vi "Run Rx - New Data.vi"(7 "New Data Support in":T1, 8 "error in (no error)":errorcluster, 10 "New Data":bool, 11 "New Data Ref":T3) -> (0 "error out":errorcluster, 5 "New Data Support out":T1)   [LabVIEW 2019, in "UDP-Custom-Device Engine.lvlib"]
uses:
  UDP-Custom-Device Engine.lvlib
  <vilib>/NI/NIVS Inline Async API/_Data Access Engine/Data Access Engine/Types/Write.DVR.ctl
  <vilib>/NI/NIVS Inline Async API/_Data Access Engine/Access Type Classes/Write/Write.lvclass
  Types/Engine - Rx New Data Options Support.ctl
  Shared/Types/Shared - New Data Options.ctl
  <vilib>/NI/NIVS Inline Async API/_Data Access Engine/Access Type Classes/Write/Write.lvclass/Write.ctl
  <vilib>/NI/NIVS Inline Async API/_Data Access Engine/Data Access Engine/Methods/Write.Data.vi
  <vilib>/NI/NIVS Inline Async API/_Data Access Engine/Access Type Classes/Write/Write.ProcessData.vi
  <vilib>/NI/NIVS Inline Async API/_Data Access Engine/Data Access Engine/Data Access Engine.lvclass
  Shared/UDP-Custom-Device Shared.lvlib
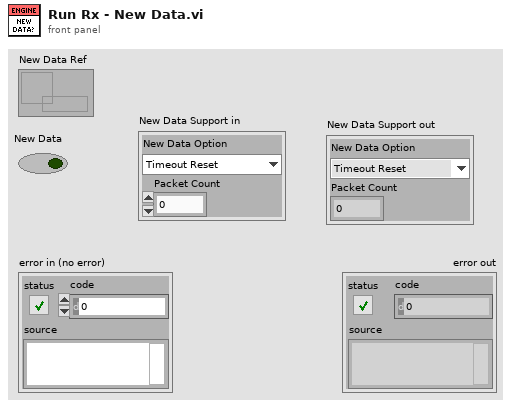
[diagram p1: front panel]
types:
  T1 = typedef "UDP-Custom-Device Engine.lvlib/Engine - Rx New Data Options Support.ctl" = cluster{"New Data Option":T2, "Packet Count":dbl}
  T2 = typedef "UDP-Custom-Device Shared.lvlib/Shared - New Data Options.ctl" = enum16{"Timeout Reset", "Counter"}
  T3 = typedef "Data Access Engine.lvlib/Data Access Engine.lvclass/Write.DVR.ctl" = refnum<data-value>
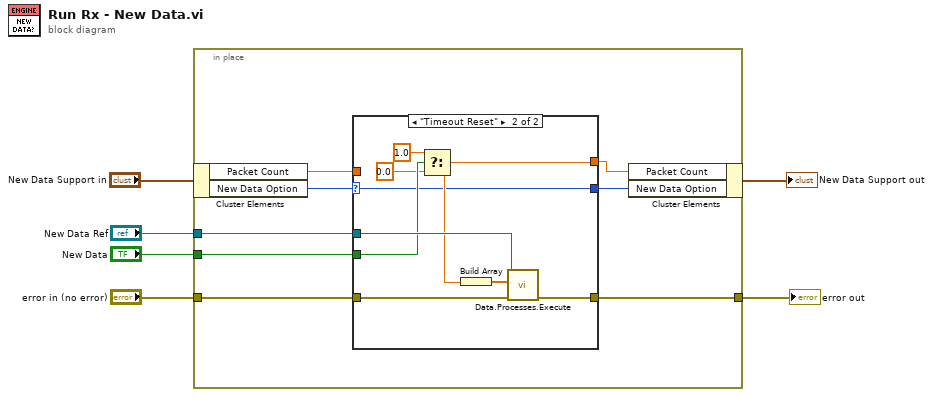
[diagram p0: block diagram]
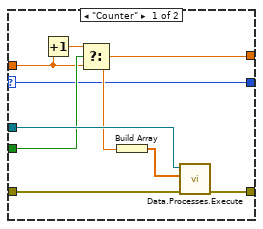
[diagram p2: hidden frame]
diagram:
  n1 = in-place {
    in-place-border: "error in (no error)" -> [w14]
    in-place-border: [w13] -> w5
    in-place-border: "New Data Ref" -> [w12]
    in-place-border: "New Data" -> [w11]
    n2 = in-place-cluster #1("New Data Support in") -> ("Packet Count"=w9:dbl, "New Data Option"=w10:T2)
    n3 = case shown="\"Timeout Reset\"" w10 {
      selector: w10 -> [w15 w24]
      tunnel: w14 -> [w22 w31]
      tunnel: [w21 w30] -> w13
      tunnel: w12 -> [w20 w29]
      tunnel: w11 -> [w19 w28]
      tunnel: [w17 w27] -> w8
      tunnel: w9 -> [w16 _]
      tunnel: [w15 w24] -> w7
      frame "Counter" {
        n4 = Increment(x=w16) -> (x+1=w18:dbl)
        n5 = Select(t=w18, s=w19, f=w16) -> (s? t:f=w17:dbl)
        n6 = Build Array(w17) -> (w23:dbl[])
        n7 = call-poly <vilib>:"Data.Processes.Execute.vi"("error in (no error)"=w22, "Values"=w23, "Ref"=w20) -> ("error out"=w21:errorcluster)  [unwired: 8 in]
      }
      frame "Timeout Reset" {
        n8 = Select(t=1.0 ("Packet Count in"), s=w28, f=0.0 ("Packet Count in")) -> (s? t:f=w27:dbl)
        n9 = Build Array(w27) -> (w32:dbl[])
        n10 = call-poly <vilib>:"Data.Processes.Execute.vi"("error in (no error)"=w31, "Values"=w32, "Ref"=w29) -> ("error out"=w30:errorcluster)  [unwired: 8 in]
      }
    }
    n11 = in-place-cluster #1("Packet Count"=w8, "New Data Option"=w7) -> (→"New Data Support out":T1)
  }
  "error out" <- w5
